vi "Tree_ItemArrayTag_Tests.vi"(11 "error in":errorcluster) -> (15 "error out":errorcluster)   [LabVIEW 2016, in "DronaTest.lvlib"]
uses:
  DronaTest.lvlib
  APIs/Stimulus/ControlValue/SetValueAuto.vi
  APIs/Stimulus/ControlValue/Controls/Tree/SetValueByItemTagArray.vi
  APIs/Assert/AssertControlValue/Equal.vi
  <vilib>/addons/_JKI Toolkits/Caraya/classes/Test/Test.lvclass
  Drona.lvlib
  <vilib>/SLL Toolkit/SLL Debug/SLL Debug.lvlib
  APIs/Assert/AssertControlValue/AssertControlValue.lvlib
  APIs/Stimulus/ControlValue/ControlValue.lvlib
  <vilib>/addons/_JKI Toolkits/Caraya/classes/Assert/Assert.lvclass
  APIs/Stimulus/ControlValue/Controls/Tree/StimulusTree.lvlib
  APIs/Get/GetControlRef/GetControlRef.lvlib
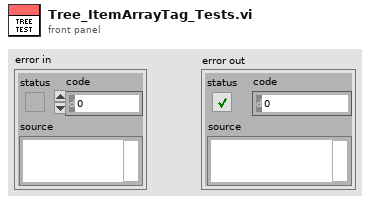
[diagram p1: front panel]
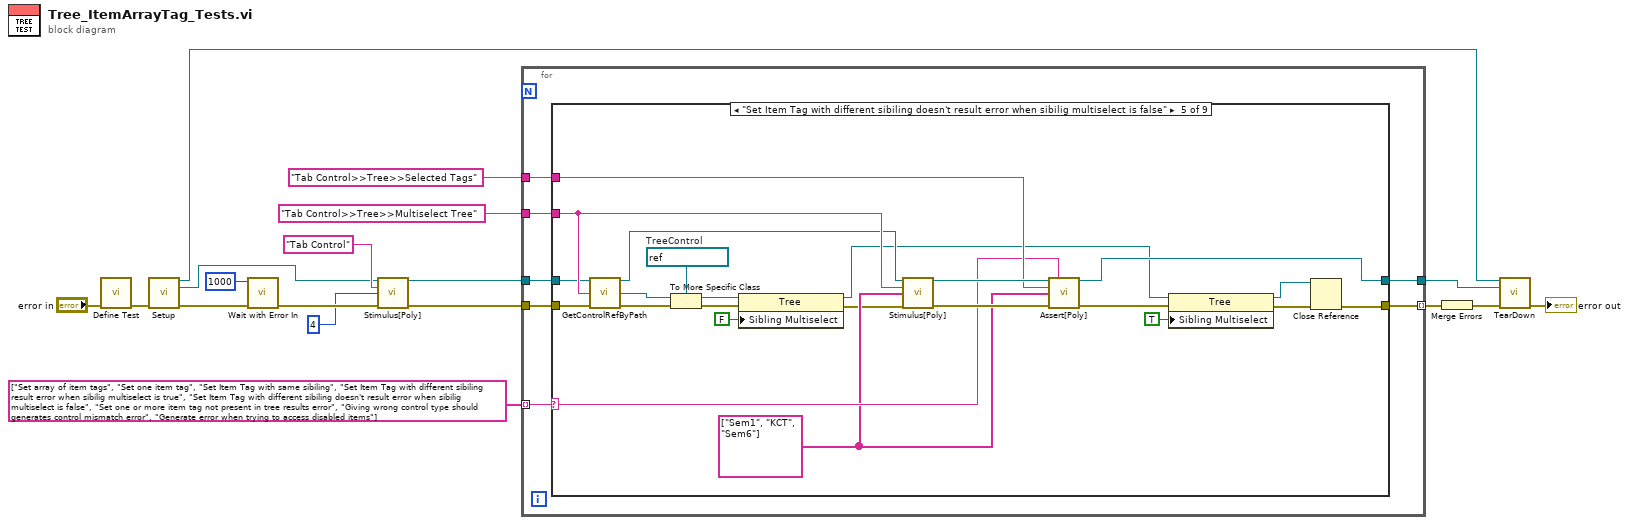
[diagram p0: block diagram]
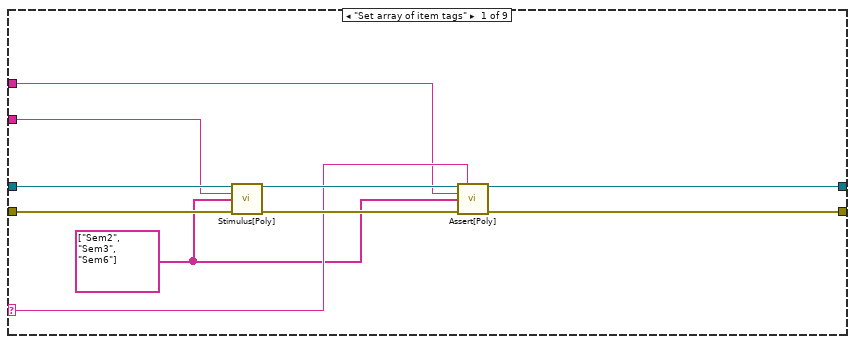
[diagram p2: hidden frame]
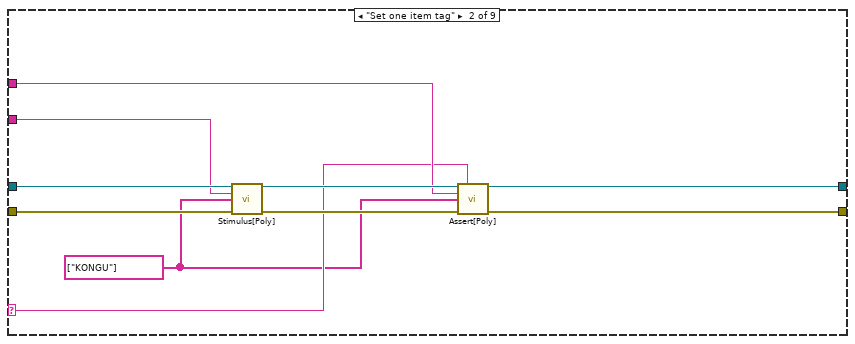
[diagram p3: hidden frame]
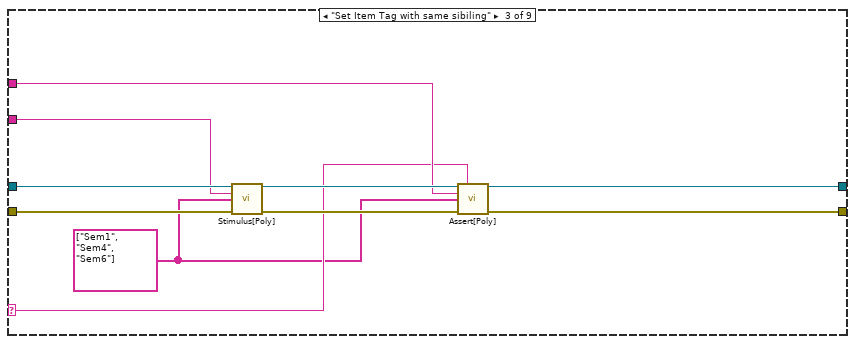
[diagram p4: hidden frame]
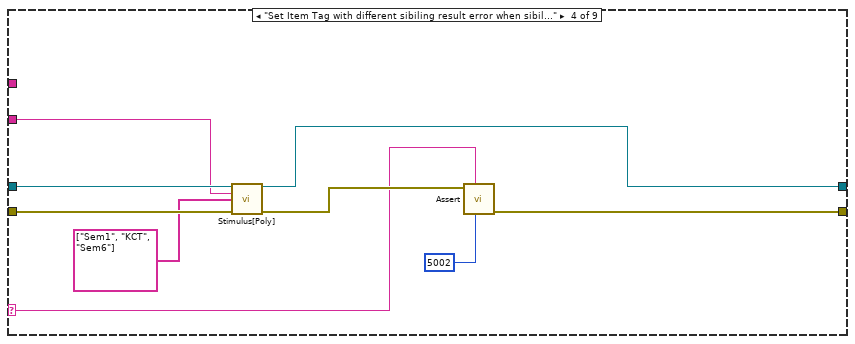
[diagram p5: hidden frame]
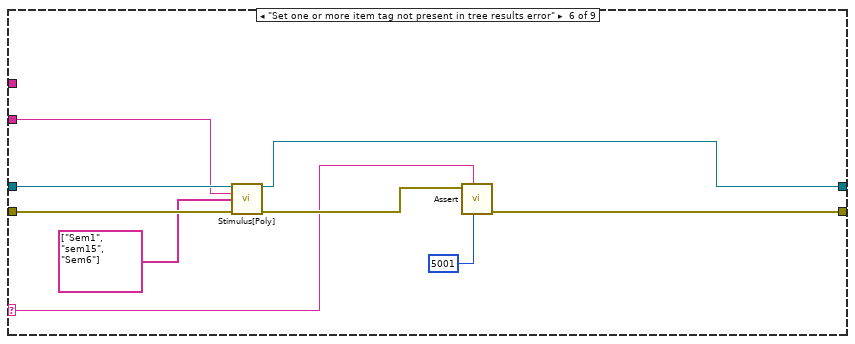
[diagram p6: hidden frame]
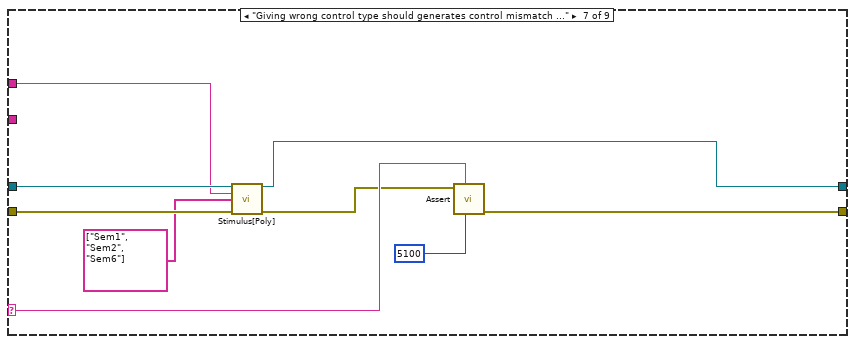
[diagram p7: hidden frame]
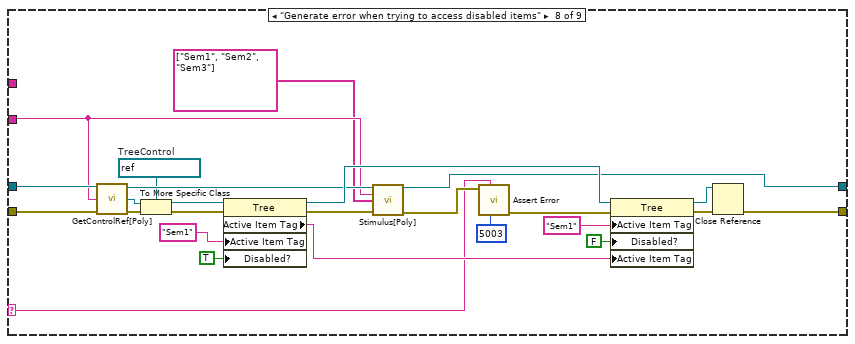
[diagram p8: hidden frame]
diagram:
  n1 = call <vilib>:"Define Test.vi"("error in (no error)"="error in") -> ("error out"=w7:errorcluster)  [unwired: 9 in, 1 out]
  n2 = call "Setup.vi"("error in (no error)"=w7) -> ("Application Ref"=w2:refnum<vi>, "VI out"=w6:refnum<vi>, "error out"=w5:errorcluster)  [unwired: 12 in]
  n3 = call <vilib>:"Wait with Error In.vi"("error in (no error)"=w5, "milliseconds to wait"=u32 1000) -> ("error out"=w16:errorcluster)  [unwired: 9 in]
  n4 = call-poly "Stimulus[Poly].vi"("VI Reference In"=w6, "Control Path"="Tab Control", "Value (Signaling)"=4, "error in"=w16) -> ("VI Reference Out"=w12:refnum<vi>, "error out"=w15:errorcluster)  [unwired: 10 in]
  n5 = for {
    tunnel: w12 -> [w24]
    tunnel: "Tab Control>>Tree>>Multiselect Tree" ("Control Path") -> [w23]
    tunnel: "Tab Control>>Tree>>Selected Tags" ("Control Path") -> [w22]
    tunnel: string[] ["Set array of item tags", "Set one item tag", "Set Item Tag with same sibiling", "Set Item Tag with different sibiling result error when sibilig multiselect is true", "Set Item Tag with different sibiling doesn't result error when sibilig multiselect is false", "Set one or more item tag not present in tree results error", "Giving wrong control type should generates control mismatch error", "Generate error when trying to access disabled items"] -> [w20] mode=indexing
    tunnel: [w19] -> w3
    tunnel: w15 -> [w25]
    tunnel: [w21] -> w8 mode=indexing
    n6 = case shown="\"Set Item Tag with different sibiling doesn't result error when sibilig multiselect is false\"" w20 {
      selector: w20 -> [w29 w37 w47 w59 w83 w90 w102 w107 _]
      tunnel: w25 -> [w35 w45 w55 w64 w81 w96 w105 w112 w132]
      tunnel: w24 -> [w34 w44 w54 w63 w79 w95 w104 w111 w131]
      tunnel: w23 -> [w27 w41 w51 w62 w80 w94 _ w110 _]
      tunnel: w22 -> [w28 w40 w50 _ w85 _ w98 _ _]
      tunnel: [w31 w39 w49 w57 w66 w93 w103 w109 w132] -> w21
      tunnel: [w30 w38 w48 w56 w84 w92 w101 w108 w131] -> w19
      frame "Set array of item tags" {
        w26 = string[] ["Sem2", "Sem3", "Sem6"] ("Item Name")
        n7 = call-poly "Stimulus[Poly].vi"("VI Reference In"=w34, "Control Path"=w27, "Item Tags Array"=w26, "Error In"=w35) -> ("VI Reference Out"=w32:refnum<vi>, "Error Out"=w33:errorcluster)  [unwired: 10 in]
        n8 = call-poly "Assert[Poly].vi"("VI Reference In"=w32, "Test Label"=w29, "Control Path"=w28, "Control Value"=w26, "Error In"=w33) -> ("VI Reference Out"=w30:refnum<vi>, "Error Out"=w31:errorcluster)  [unwired: 8 in, 1 out]
      }
      frame "Set one item tag" {
        w36 = string[] ["KONGU"] ("Item Name")
        n9 = call-poly "Stimulus[Poly].vi"("VI Reference In"=w44, "Control Path"=w41, "Item Tags Array"=w36, "Error In"=w45) -> ("VI Reference Out"=w42:refnum<vi>, "Error Out"=w43:errorcluster)  [unwired: 10 in]
        n10 = call-poly "Assert[Poly].vi"("VI Reference In"=w42, "Test Label"=w37, "Control Path"=w40, "Control Value"=w36, "Error In"=w43) -> ("VI Reference Out"=w38:refnum<vi>, "Error Out"=w39:errorcluster)  [unwired: 8 in, 1 out]
      }
      frame "Set Item Tag with same sibiling" {
        w46 = string[] ["Sem1", "Sem4", "Sem6"] ("Item Name")
        n11 = call-poly "Stimulus[Poly].vi"("VI Reference In"=w54, "Control Path"=w51, "Item Tags Array"=w46, "Error In"=w55) -> ("VI Reference Out"=w52:refnum<vi>, "Error Out"=w53:errorcluster)  [unwired: 10 in]
        n12 = call-poly "Assert[Poly].vi"("VI Reference In"=w52, "Test Label"=w47, "Control Path"=w50, "Control Value"=w46, "Error In"=w53) -> ("VI Reference Out"=w48:refnum<vi>, "Error Out"=w49:errorcluster)  [unwired: 8 in, 1 out]
      }
      frame "Set Item Tag with different sibiling result error when sibilig multiselect is true" {
        n13 = call-poly "Stimulus[Poly].vi"("VI Reference In"=w63, "Control Path"=w62, "Item Tags Array"=string[] ["Sem1", "KCT", "Sem6"] ("Item Name"), "Error In"=w64) -> ("VI Reference Out"=w56:refnum<vi>, "Error Out"=w60:errorcluster)  [unwired: 10 in]
        n14 = call-poly <vilib>:"Assert.vi"("error code (1)"=5002, "Label"=w59, "Error?"=w60) -> ("error out"=w57:errorcluster)  [unwired: 7 in, 1 out]
      }
      frame "Set Item Tag with different sibiling doesn't result error when sibilig multiselect is false" {
        w75 = refnum<vi> refnum  # TreeControl
        w82 = string[] ["Sem1", "KCT", "Sem6"] ("Item Name")
        n15 = call "GetControlRefByPath.vi"("VI Reference In"=w79, "Control Path"=w80, "error In"=w81) -> ("VI Reference Out"=w78:refnum<vi>, "Ctl Refnum"=w77:refnum<vi>, "error out"=w76:errorcluster)  [unwired: 10 in]
        n16 = To More Specific Class(target class=w75, reference=w77, error in=w76) -> (specific class reference=w74:refnum<vi>, error out=w73:errorcluster)
        n17 = property class="Tree"(reference=w74, error in=w73, "Sibling Multiselect"=FALSE) -> (reference out=w67:refnum<vi>, error out=w71:errorcluster)
        n18 = call-poly "Stimulus[Poly].vi"("VI Reference In"=w78, "Control Path"=w80, "Item Tags Array"=w82, "Error In"=w71) -> ("VI Reference Out"=w86:refnum<vi>, "Error Out"=w87:errorcluster)  [unwired: 10 in]
        n19 = call-poly "Assert[Poly].vi"("VI Reference In"=w86, "Test Label"=w83, "Control Path"=w85, "Control Value"=w82, "Error In"=w87) -> ("VI Reference Out"=w84:refnum<vi>, "Error Out"=w69:errorcluster)  [unwired: 8 in, 1 out]
        n20 = property class="Tree"(reference=w67, error in=w69, "Sibling Multiselect"=TRUE) -> (reference out=w65:refnum<vi>, error out=w68:errorcluster)
        n21 = Close Reference(reference=w65, error in (no error)=w68) -> (error out=w66:errorcluster)
      }
      frame "Set one or more item tag not present in tree results error" {
        n22 = call-poly "Stimulus[Poly].vi"("VI Reference In"=w95, "Control Path"=w94, "Item Tags Array"=string[] ["Sem1", "sem15", "Sem6"] ("Item Name"), "Error In"=w96) -> ("VI Reference Out"=w92:refnum<vi>, "Error Out"=w91:errorcluster)  [unwired: 10 in]
        n23 = call-poly <vilib>:"Assert.vi"("error code (1)"=5001, "Label"=w90, "Error?"=w91) -> ("error out"=w93:errorcluster)  [unwired: 7 in, 1 out]
      }
      frame "Giving wrong control type should generates control mismatch error" {
        n24 = call-poly "Stimulus[Poly].vi"("VI Reference In"=w104, "Control Path"=w98, "Item Tags Array"=string[] ["Sem1", "Sem2", "Sem6"] ("Item Name"), "Error In"=w105) -> ("VI Reference Out"=w101:refnum<vi>, "Error Out"=w100:errorcluster)  [unwired: 10 in]
        n25 = call-poly <vilib>:"Assert.vi"("error code (1)"=5100, "Label"=w102, "Error?"=w100) -> ("error out"=w103:errorcluster)  [unwired: 7 in, 1 out]
      }
      frame "Generate error when trying to access disabled items" {
        w116 = refnum<vi> refnum  # TreeControl
        n26 = call-poly "GetControlRef[Poly].vi"("VI Reference In"=w111, "Control Path"=w110, "error In"=w112) -> ("VI Reference Out"=w123:refnum<vi>, "Ctl Refnum"=w115:refnum<vi>, "error out"=w113:errorcluster)  [unwired: 10 in]
        n27 = To More Specific Class(target class=w116, reference=w115, error in=w113) -> (specific class reference=w117:refnum<vi>, error out=w114:errorcluster)
        n28 = property class="Tree"(reference=w117, error in=w114, "Active Item Tag"="Sem1" ("Active Item:Tag"), "Disabled?"=TRUE ("Active Item:Disabled?")) -> (reference out=w127:refnum<vi>, error out=w122:errorcluster, "Active Item Tag"=w128:string)
        n29 = call-poly "Stimulus[Poly].vi"("VI Reference In"=w123, "Control Path"=w110, "Item Tags Array"=string[] ["Sem1", "Sem2", "Sem3"], "Error In"=w122) -> ("VI Reference Out"=w108:refnum<vi>, "Error Out"=w124:errorcluster)  [unwired: 10 in]
        n30 = call <vilib>:"Assert Error.vi"("error code (1)"=5003, "Label"=w107, "Error?"=w124) -> ("error out"=w125:errorcluster)  [unwired: 7 in, 1 out]
        n31 = property class="Tree"(reference=w127, error in=w125, "Active Item Tag"="Sem1" ("Active Item:Tag"), "Disabled?"=FALSE ("Active Item:Disabled?"), "Active Item Tag"=w128) -> (reference out=w121:refnum<vi>, error out=w120:errorcluster)
        n32 = Close Reference(reference=w121, error in (no error)=w120) -> (error out=w109:errorcluster)
      }
      frame Default {
      }
    }
  }
  n33 = Merge Errors(w8) -> (w4:errorcluster)
  n34 = call "TearDown.vi"("Application Ref"=w2, "VI in"=w3, "error in (no error)"=w4) -> ("error out"=→"error out":errorcluster)  [unwired: 12 in]
